vi "Write ini Array.vi"(0 "configuration file path":path, 5 "section":string, 7 "KeysArray":string[](array[string]), 9 "ValueArray":dbl[](array[numeric]), 11 "error in (no error)":errorcluster) -> (15 "error out":errorcluster)   [LabVIEW 2015]
uses:
  <vilib>/Utility/config.llb/Write Key (Double).vi
  <vilib>/Utility/config.llb/NI_LVConfig.lvlib
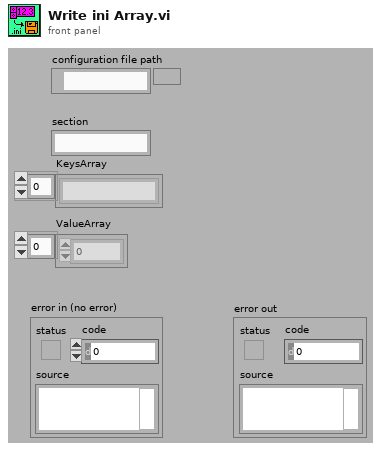
[diagram p1: front panel]
types:
  T1 = typedef "NI_LVConfig.lvlib/Config Data RefNum.ctl" = refnum<k1>
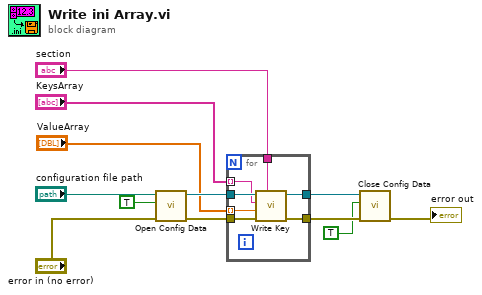
[diagram p0: block diagram]
diagram:
  n1 = call <vilib>:"Open Config Data.vi"("error in (no error)"="error in (no error)", "create file if necessary (T)"=TRUE ("create file if necessary? (T)"), "configuration file path"="configuration file path") -> ("error out"=w7:errorcluster, "refnum"=w8:T1)  [unwired: 6 in, 1 out]
  n2 = for {
    tunnel: "section" -> [w19]
    tunnel: w8 -> [w18]
    tunnel: w7 -> [w17]
    tunnel: [w16] -> w6
    tunnel: [w15] -> w5
    tunnel: "KeysArray" -> [w14] mode=indexing
    tunnel: "ValueArray" -> [w13] mode=indexing
    n3 = call-poly <vilib>:"Write Key.vi"("section"=w19, "error in (no error)"=w17, "value"=w13, "key"=w14, "refnum"=w18) -> ("error out"=w15:errorcluster, "refnum out"=w16:T1)  [unwired: 4 in, 1 out]
  }
  n4 = call <vilib>:"Close Config Data.vi"("error in (no error)"=w5, "write file if changed (T)"=TRUE ("write configuration file? (T)"), "refnum"=w6) -> ("error out"=→"error out":errorcluster)  [unwired: 7 in, 1 out]
